vi "Teleop Storage Controls.vi"(8 "Call Context":T1, 10 "Store Button":bool, 11 "Storing Can?":bool) -> (2 "Store Can?":bool)   [LabVIEW 2014]
uses:
  <vilib>/Rock Robotics/WPI/DriverStation/WPI_DriverStationDerivedRobotMode.ctl
  Common Code/Change Detect Boolean.vi
  Common Code/Change Detect Int.vi
  Robot Global Data.vi
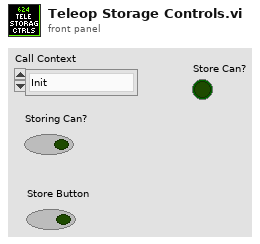
[diagram p1: front panel]
types:
  T1 = typedef "WPI_DriverStationDerivedRobotMode.ctl" = enum16{"Init", "Execute", "Stop"}
  T2 = typedef "Elevator Mode.ctl" = enum16{"Manual", "Safe", "Auto"}
  T3 = typedef "Elevator Status.ctl" = cluster{"Height":dbl, "Enc Value":dbl, "Limit Override":bool, "Mode":T2, "High IR":bool, "Motor Out":dbl, "Ping Detect":bool, "Auto Elevator Indicators":T4, "Master Current":dbl, "Slave Current":dbl, "High Current":bool, "Current Tripped":bool, "Top Limit":bool, "Bottom Limit":bool, "Eject Piston":bool, "Stabilizer":bool, "Finger":bool, "Finger Height":dbl, "Finger Raw":dbl, "Finger at Bottom":bool}
  T4 = typedef "Auto Elevator Indicators.ctl" = cluster{"Target Out":dbl, "Storing Trashcan?":bool, "State":T5, "In Range":bool, "Store Can Command":bool, "HP Load":bool}
  T5 = typedef "Elevator State.ctl" = enum16{"Idle", "Goto Load Position", "Wait for Load", "Load Drop", "Load Lift", "Drop Stack", "Goto Eject Position", "Eject ", "Raise Trashcan", "Open Stabilizer", "Untip Drop", "Untip Wait", "Untip Lift", "Abort Load", "HP Load Wait", "HP Load Drop", "HP Load Lift", "HP Load Abort", "Close Stabilizer", "HP Load Unfinish", "HP Load Score", "HP Load Finish", "HP Goto Finish Down", "HP Goto Finish Up"}
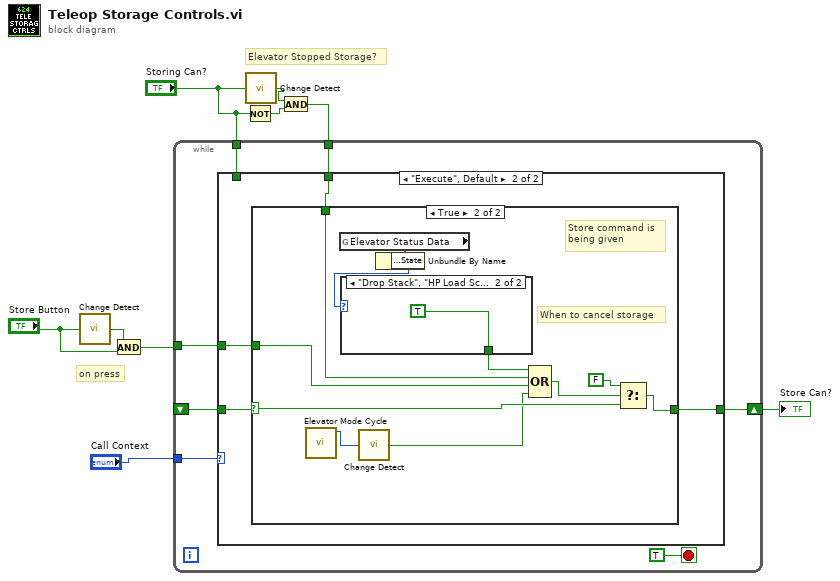
[diagram p0: block diagram]
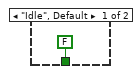
[diagram p4: hidden frame]
diagram:
  # "on press"
  # "Elevator Stopped Storage?"
  n1 = call-poly "Change Detect.vi"("In"="Store Button") -> ("Changed?"=w5:bool)
  n2 = And(x=w5, y="Store Button") -> (x .and. y?=w3:bool)
  n3 = Not(x="Storing Can?") -> (.not. x?=w9:bool)
  n4 = call-poly "Change Detect.vi"("In"="Storing Can?") -> ("Changed?"=w8:bool)
  n5 = And(x=w8, y=w9) -> (x .and. y?=w7:bool)
  n6 = while {
    shift-right: [w13] -> w6
    shift-left: _ -> [w15]
    tunnel: w7 -> [w14]
    tunnel: w3 -> [w12]
    tunnel: "Call Context" -> [w11]
    tunnel: "Storing Can?" -> [w10]
    stop <- TRUE stop-if-true
    n7 = case shown="\"Execute\", Default" w11 {
      tunnel: w15 -> [_ w21]
      tunnel: w14 -> [_ w20]
      tunnel: [w17 w19] -> w13
      tunnel: w12 -> [_ w18]
      tunnel: w10 -> [w17 _]
      frame "Init" {
        # "First call of teleop after autonomous\nremember what elevator is storing"
      }
      frame "Execute", Default {
        n8 = case shown="True" w21 {
          selector: w21 -> [_ w32]
          tunnel: w20 -> [_ w30]
          tunnel: [w22 w31] -> w19
          tunnel: w18 -> [w22 w28]
          frame False {
            # "Store command not being given"
            # "start store on press"
          }
          frame True {
            # "Store command is\nbeing given"
            # "When to cancel storage"
            n9 = call "Elevator Mode Cycle.vi"() -> ("Mode"=w24:T2)  [unwired: 11 in]
            n10 = global read "Robot Global Data.vi" "Elevator Status Data"() -> (w27:T3)
            n11 = call-poly "Change Detect.vi"("In"=w24) -> ("Changed?"=w23:bool)
            n12 = Unbundle By Name(w27) -> ("Auto Elevator Indicators.State"=w26:T5)
            n13 = case shown="\"Drop Stack\", \"HP Load Score\"" w26 {
              tunnel: [FALSE TRUE] -> w25
              frame "Idle", Default {
              }
              frame "Drop Stack", "HP Load Score" {
              }
            }
            n14 = Compound Arithmetic op=OR(w25, w30, w28, w23) -> (w29:bool)
            n15 = Select(t=FALSE, s=w29, f=w32) -> (s? t:f=w31:bool)
          }
        }
      }
    }
  }
  "Store Can?" <- w6
